vi "Message Callbacks.vi"(8 "error in (no error)":errorcluster, 10 "Message ID":string, 11 "Manager in":refnum<class "Manager.lvclass">) -> (0 "error out":errorcluster, 2 "Callbacks":T1[](array[typedef]), 3 "Manager out":refnum<class "Manager.lvclass">)   [LabVIEW 2020, in "Stream-Simple-Msg.lvlib" / "Manager.lvclass"]
uses:
  Manager.lvclass
  Callback.ctl
  Message/Message.lvclass
  Manager.lvclass/Manager.ctl
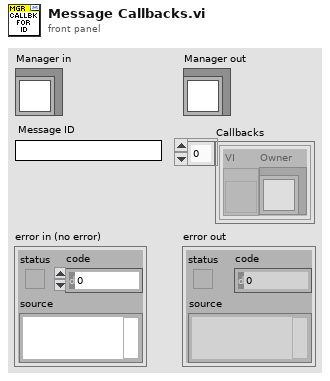
[diagram p1: front panel]
types:
  T1 = typedef "Stream-Simple-Msg.lvlib/Manager.lvclass/Callback.ctl" = cluster{"VI":refnum<vi>, "Owner":refnum<class>}
  T2 = typedef "Stream-Simple-Msg.lvlib/Manager.lvclass/Ref Data.ctl" = cluster{"Message Callbacks":map{string, T1[]}, "Endpoints":map{string, refnum<class "Endpoint.lvclass">}, "Stream Endpoints":refnum<class "Endpoint.lvclass">[], "State Callbacks":T3[]}
  T3 = typedef "Stream-Simple-Msg.lvlib/Manager.lvclass/State Callback.ctl" = cluster{"Owner":refnum<class>, "VI":refnum<vi>}
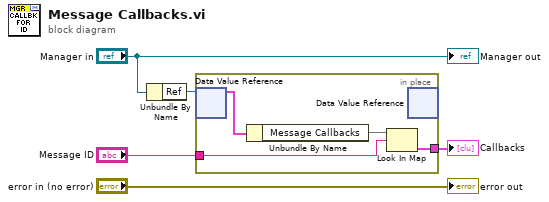
[diagram p0: block diagram]
diagram:
  n1 = Unbundle By Name("Manager in") -> ("Ref"=w3:refnum<data-value>)
  n2 = in-place {
    in-place-border: [w7] -> w1
    in-place-border: "Message ID" -> [w6]
    n3 = in-place-dvr #1(w3) -> (w9:T2)  [unwired: 1 out]
    n4 = Unbundle By Name(w9) -> ("Message Callbacks"=w8:map{string, T1[]})
    n5 = Look In Map(map=w8, key=w6) -> (value=w7:T1[])  [unwired: 1 in, 1 out]
    n6 = in-place-dvr #1() -> ()  [unwired: 1 in, 2 out]
  }
  "Callbacks" <- w1
  "error out" <- "error in (no error)"
  "Manager out" <- "Manager in"
